vi "handle user check.vi"(8 "error in (no error)":errorcluster, 11 "REF":T1) -> (0 "error out":errorcluster, 2 "Result":bool, 3 "REF out":T1)   [LabVIEW 2024]
uses:
  CTRLS/REF.ctl
  CTRLS/Main Tabs.ctl
  CTRLS/Open Batch Data.ctl
  CTRLS/DM_Data.ctl
  CTRLS/run statistics.ctl
  CTRLS/System settings.ctl
  CTRLS/Printer Message settings.ctl
  CTRLS/DB operation Selector.ctl
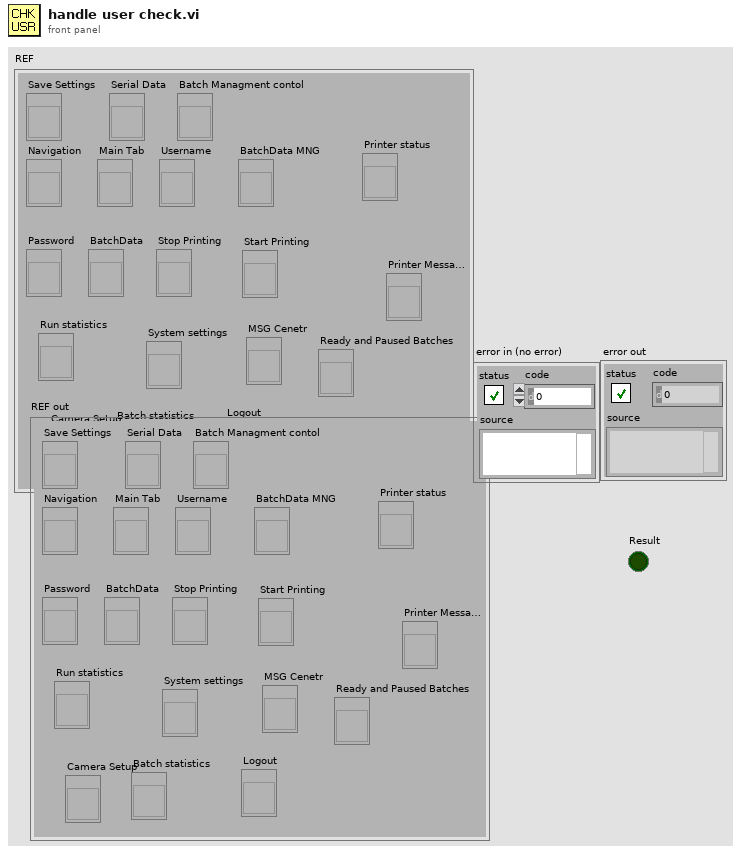
[diagram p1: front panel]
types:
  T1 = typedef "REF.ctl" = cluster{"Save Settings":refnum<vi>, "Navigation":refnum<vi>, "Main Tab":refnum<vi>, "Password":refnum<vi>, "BatchData":refnum<vi>, "Serial Data":refnum<vi>, "Username":refnum<vi>, "Stop Printing":refnum<vi>, "Run statistics":refnum<vi>, "System settings":refnum<vi>, "Batch Managment contol":refnum<vi>, "Start Printing":refnum<vi>, "BatchData MNG":refnum<vi>, "MSG Cenetr":refnum<vi>, "Printer status":refnum<vi>, "Printer Message Config":refnum<vi>, "Ready and Paused Batches":refnum<vi>, "Camera Setup":refnum<vi>, "Batch statistics":refnum<vi>, "Logout":refnum<vi>}
  T2 = typedef "DB operation Selector.ctl" = enum16{"Select", "Insert", "Update", "Execute select Query", "Execute update query"}
  T3 = typedef "NI_Database_API.lvlib/Conn ObjectReference.ctl" = refnum<k1>
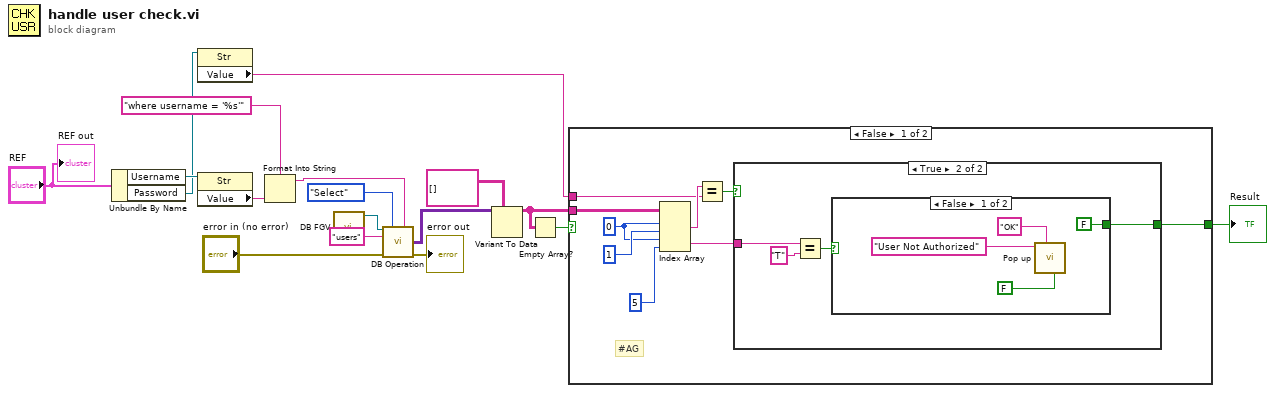
[diagram p0: block diagram]
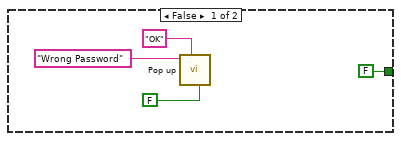
[diagram p2: hidden frame]
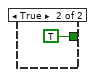
[diagram p3: hidden frame]
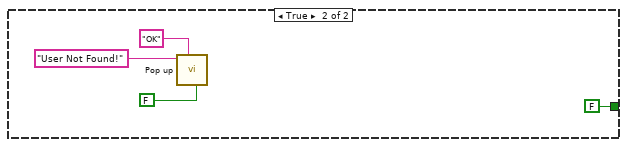
[diagram p4: hidden frame]
diagram:
  n1 = Unbundle By Name("REF") -> ("Username"=w16:refnum<vi>, "Password"=w15:refnum<vi>)
  n2 = property class="Str"(reference=w15) -> ("Value"=w3:string)  [unwired: 1 in, 2 out]
  n3 = property class="Str"(reference=w16) -> ("Value"=w10:string)  [unwired: 1 in, 2 out]
  n4 = Format Into String(format string="where username = '%s'" ("Condition"), w10) -> (resulting string=w9:string)  [unwired: 2 in, 1 out]
  n5 = call "DB FGV.vi"() -> ("DB ref"=w14:T3)  [unwired: 11 in]
  n6 = call "DB Operation.vi"("connection reference"=w14, "DB Op Selector"=DB_operation_Selector."Select", "Condition"=w9, "table"="users", "error in (no error)"="error in (no error)") -> ("data out"=w7:variant[][], "error out"=→"error out":errorcluster)  [unwired: 8 in, 1 out]
  n7 = Variant To Data(type=string[][] [], Variant=w7) -> (data=w4:string[][])  [unwired: 1 in, 1 out]
  n8 = Empty Array?(array=w4) -> (empty?=w6:bool)
  n9 = case shown="False" w6 {
    tunnel: [w21 FALSE] -> w5
    tunnel: w4 -> [w26 _]
    tunnel: w3 -> [w23 _]
    frame False {
      w20 = 0 ("disabled index (row)")
      # "#AG"
      n10 = Index Array(array=w26, index (row) #1=w20, index (col) #1=1 ("disabled index (col)"), index (row) #2=w20, index (col) #2=5 ("disabled index (col)")) -> (element #1=w24:string, element #2=w18:string)
      n11 = Equal?(x=w24, y=w23) -> (x = y?=w22:bool)
      n12 = case shown="True" w22 {
        tunnel: [FALSE w31] -> w21
        tunnel: w18 -> [_ w34]
        frame False {
          n13 = call "Pop up.vi"("Close Visible"=FALSE, "OK Boolean Text"="OK", "Title IN"="Wrong Password") -> ()  [unwired: 7 in, 2 out]
        }
        frame True {
          n14 = Equal?(x=w34, y="T") -> (x = y?=w32:bool)
          n15 = case shown="False" w32 {
            tunnel: [FALSE TRUE] -> w31
            frame False {
              n16 = call "Pop up.vi"("Close Visible"=FALSE, "OK Boolean Text"="OK", "Title IN"="User Not Authorized") -> ()  [unwired: 7 in, 2 out]
            }
            frame True {
            }
          }
        }
      }
    }
    frame True {
      n17 = call "Pop up.vi"("Close Visible"=FALSE, "OK Boolean Text"="OK", "Title IN"="User Not Found!") -> ()  [unwired: 7 in, 2 out]
    }
  }
  "Result" <- w5
  "REF out" <- "REF"
